vi "Record Continuous Tags v2.0.0.vi"(0 "Record \"Num_Blocks\"":bool=TRUE caption="Disable", 1 "Num_Blocks":dbl=13.0, 5 "Data Tag":dbl format="%.2p", 6 "Waveform Array In":waveform(dbl)[](array[waveform]), 7 "TDMS Props":T1={"Test Cell"="TC2", "Calibration Source"="Line Driver", "Operator's Initials"="IPS", "HW Channel"="PXI1Slot3/ai0", "Sample Rate (Hz)"="10"}, 9 "Record Disable":bool caption="Record Enable", 10 "path":path=path "C:/Fuel Lab Bench Testing/Test Data/Oil Pump 171121", 13 "Main Count":dbl, 14 "Force Record":bool caption="Force Record Enable", 15 "Run Letter":string="a") -> (3 "Recorded Blocks":dbl, 4 "Record Cmd":bool, 11 "Saving Data":bool)   [LabVIEW 2017]
uses:
  <vilib>/ptbypt/NI_PtbyPt.lvlib
panel:
  out "asPropNames":string[](array[string])
  out "Main Count 2":dbl
  out "x .or. y?":bool
  in  "Data In":dbl
  out "Data Out":dbl
  in  "direction":enum16{"either", "false-true", "true-false"}(ring)=enum."false-true"
  # "Rev 131203_A, added \".lvm\" file extension to file path.\nRev 141029 adds block counter to allow fixed number of blocks recorded.\nRev 151208_A records to TDMS file type instead of the text-based \".lvm\".   This can be changed inside the \"Write to Measurement File.vi\" Express VI.\nRev 160128_A changes logic so that Force Record can override Data Tag # critieria.\nRev 161209_A prepends \"\\\" to filename so that the new file goes inside the desired directory.  This is being used initially in the Fuel Lab.\nRev 161212_A outputs number of blocks logged.\nv2.0.0 writes data to TDMS file for calibration purposes."
  # "N:\\TeamShares\\Testing Group\\Bench Tests\\PR19321 - Cooler Pressure Drop - Orthrus\\Valve PD"
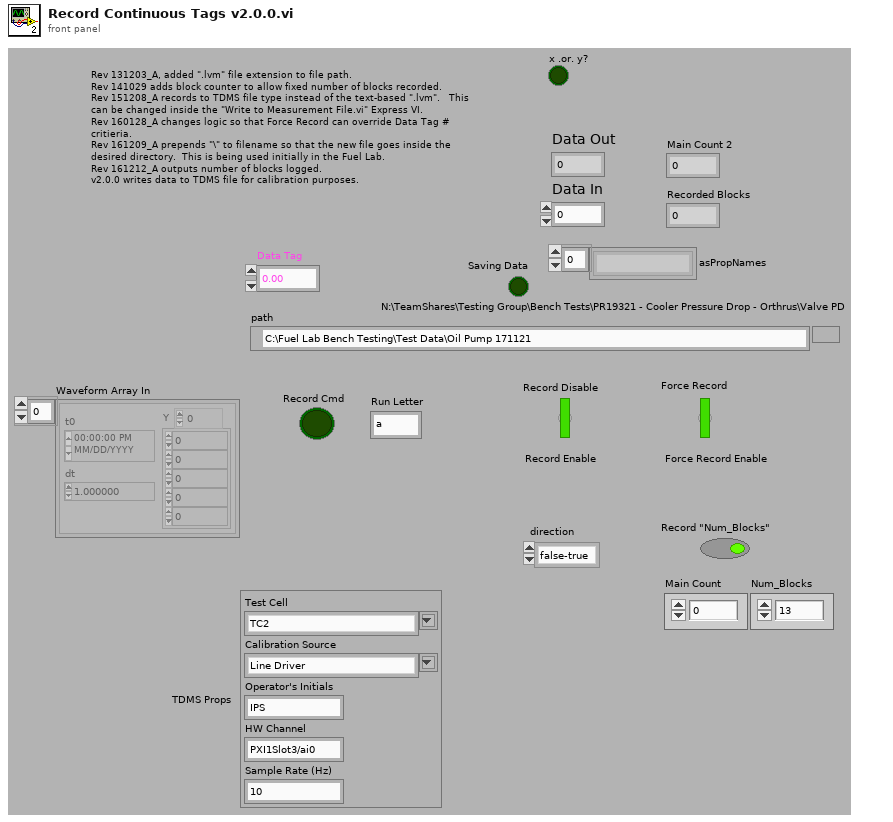
[diagram p1: front panel]
types:
  T1 = cluster{"Test Cell":string, "Calibration Source":string, "Operator's Initials":string, "HW Channel":string, "Sample Rate (Hz)":string}
  T2 = enum16{"open", "open or create", "create or replace", "create", "open (read-only)"}
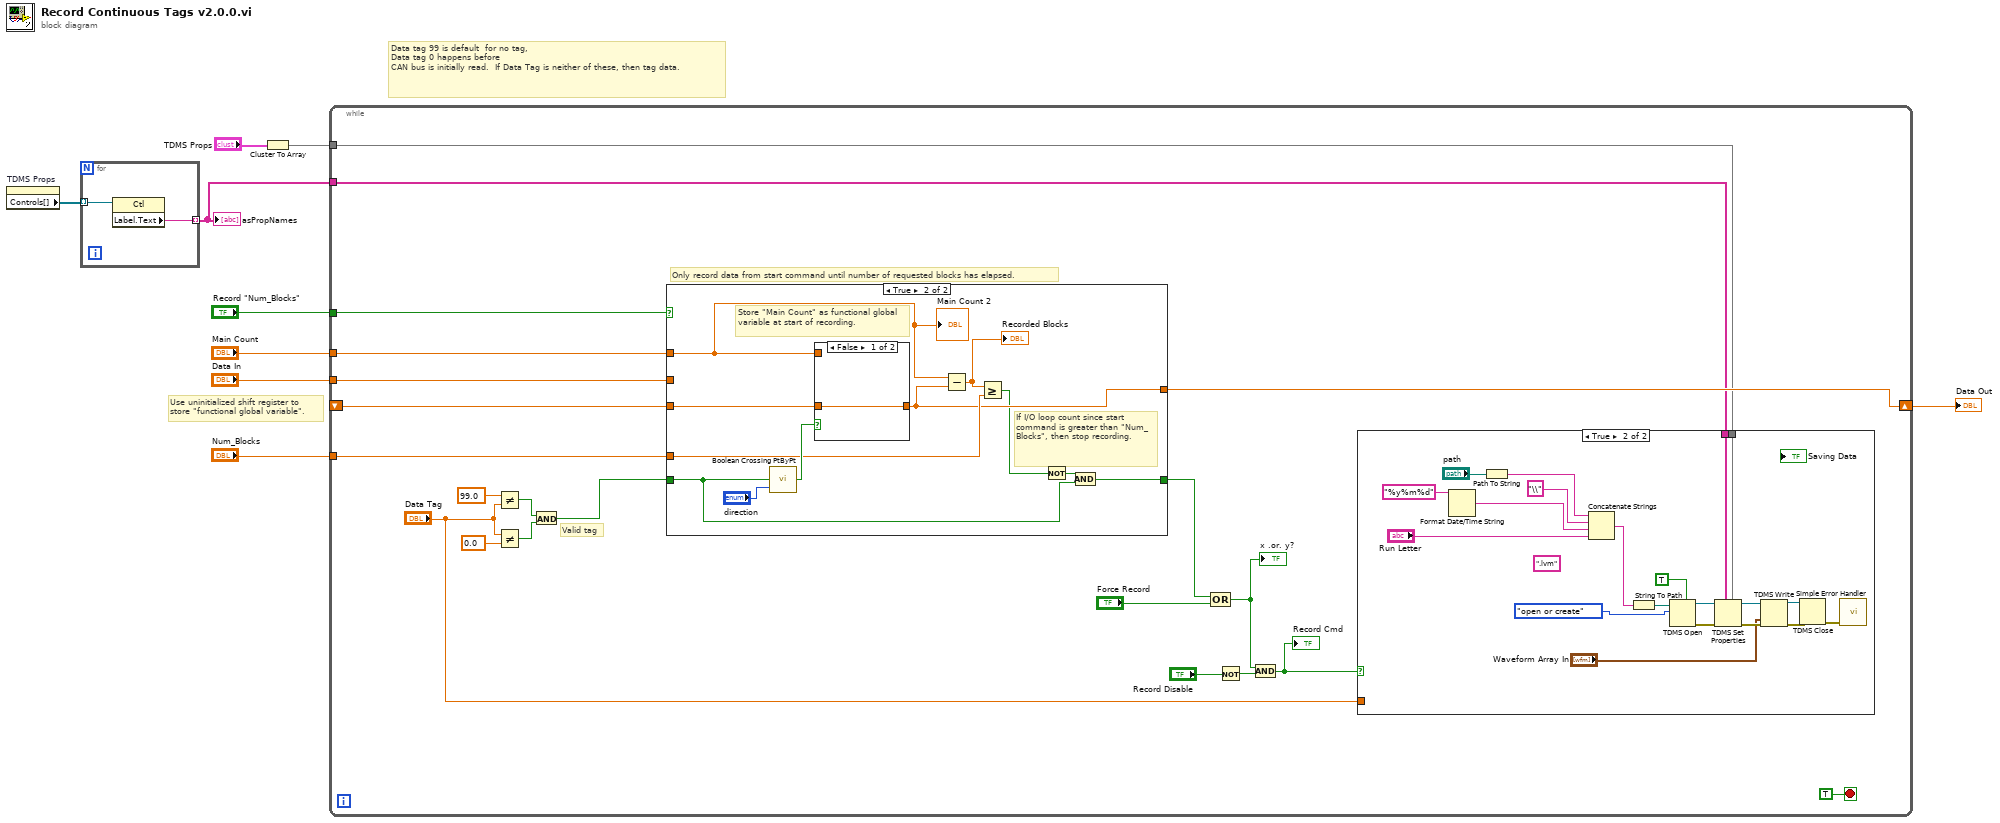
[diagram p0: block diagram]
diagram:
  # "Use uninitialized shift register to store \"functional global variable\"."
  # "Data tag 99 is default  for no tag,\nData tag 0 happens before \nCAN bus is initially read.  If Data Tag is neither of these, then tag data."
  n1 = property on="TDMS Props" class="Clust (strict)"() -> ("Controls[]"=w4:refnum<vi>[])  [unwired: 2 in, 2 out]
  n2 = for {
    tunnel: w4 -> [w11] mode=indexing
    tunnel: [w10] -> w3 mode=indexing
    n3 = property class="Ctl"(reference=w11) -> ("Label.Text"=w10:string)  [unwired: 1 in, 2 out]
  }
  "asPropNames" <- w3
  n4 = Cluster To Array(cluster="TDMS Props") -> (array=w1:string[])
  n5 = while {
    shift-right: [w17] -> w7
    shift-left: _ -> [w20]
    tunnel: "Main Count" -> [w19]
    tunnel: "Record \"Num_Blocks\"" -> [w18]
    tunnel: "Data In" -> [w16]
    tunnel: "Num_Blocks" -> [w15]
    tunnel: w1 -> [w12]
    tunnel: w3 -> [w13]
    stop <- TRUE stop-if-true
    # "Valid tag"
    # "Only record data from start command until number of requested blocks has elapsed."
    n6 = Not Equal?(x=99.0 ("y"), y="Data Tag") -> (x != y?=w24:bool)
    n7 = Not Equal?(x="Data Tag", y=0.0 ("x")) -> (x != y?=w26:bool)
    n8 = And(x=w24, y=w26) -> (x .and. y?=w23:bool)
    n9 = case shown="True" w18 {
      tunnel: w23 -> [w54 w57]
      tunnel: [w54 w58] -> w29
      tunnel: w19 -> [_ w63]
      tunnel: w15 -> [_ w62]
      tunnel: w20 -> [_ w60]
      tunnel: [w53 w59] -> w17
      tunnel: w16 -> [w53 _]
      frame False {
      }
      frame True {
        # "If I/O loop count since start command is greater than \"Num_Blocks\", then stop recording."
        # "Store \"Main Count\" as functional global variable at start of recording."
        n10 = call <vilib>:"Boolean Crossing PtByPt.vi"("direction"="direction", "input"=w57) -> ("crossing"=w64:bool)  [unwired: 1 in]
        n11 = case shown="False" w64 {
          tunnel: w63 -> [_ w67]
          tunnel: [w66 w67] -> w59
          tunnel: w60 -> [w66 _]
          frame False {
          }
          frame True {
          }
        }
        n12 = Subtract(x=w63, y=w59) -> (x-y=w61:dbl)
        "Recorded Blocks" <- w61
        n13 = Greater Or Equal?(x=w61, y=w62) -> (x >= y?=w55:bool)
        n14 = Not(x=w55) -> (.not. x?=w56:bool)
        n15 = And(x=w56, y=w57) -> (x .and. y?=w58:bool)
        "Main Count 2" <- w63
      }
    }
    n16 = Compound Arithmetic op=OR(w29, "Force Record") -> (w30:bool)
    "x .or. y?" <- w30
    n17 = Not(x="Record Disable") -> (.not. x?=w31:bool)
    n18 = And(x=w30, y=w31) -> (x .and. y?=w28:bool)
    "Record Cmd" <- w28
    n19 = case shown="True" w28 {
      tunnel: "Data Tag" -> [_ _]
      tunnel: w13 -> [_ w40]
      tunnel: w12 -> [_ w39]
      frame False {
      }
      frame True {
        (unwired) ".lvm" ("string")
        n20 = Format Date/Time String(time format string (%c)="%y%m%d" ("string")) -> (date/time string=w49:string)  [unwired: 2 out]
        n21 = Path To String(path="path") -> (string=w47:string)
        n22 = Concatenate Strings(w47, "\\" ("string"), w49, "Run Letter") -> (w48:string)
        n23 = String To Path(string=w48) -> (path=w45:path)
        n24 = TDMS Open(5:TRUE ("create index file? (T)"), 10:T2."open or create" ("operation (0:open)"), 11:w45) -> (0:w41:errorcluster, 3:w42:refnum<k34>)  [unwired: 4 in]
        n25 = TDMS Set Properties(5:w39, 7:w40, 8:w41, 11:w42) -> (0:w37:errorcluster, 3:w38:refnum<k34>)  [unwired: 2 in, 2 out]
        n26 = TDMS Write(0:w38, 9:"Waveform Array In", 11:w37) -> (4:w34:refnum<k34>, 15:w35:errorcluster)  [unwired: 3 in, 2 out]
        n27 = TDMS Close(8:w35, 11:w34) -> (0:w33:errorcluster)  [unwired: 1 out]
        n28 = call <vilib>:"Simple Error Handler.vi"("error in (no error)"=w33) -> ()  [unwired: 1 in, 8 out]
      }
    }
  }
  "Data Out" <- w7
